vi "PostRegistration.vi"(8 "error in (no error)":errorcluster, 10 "state":T1(ring), 11 "VI ref":refnum<vi>) -> (0 "error out":errorcluster, 3 "VI ref":refnum<vi>)   [LabVIEW 2021, in "Autocomplete Textbox.lvlib"]
uses:
  Autocomplete Textbox.lvlib
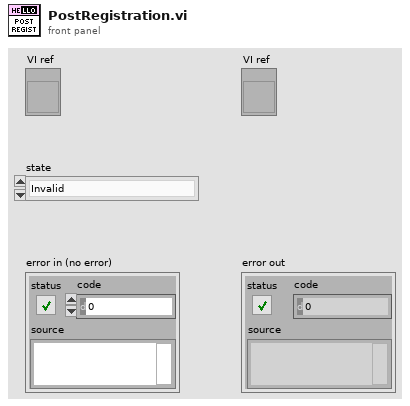
[diagram p1: front panel]
types:
  T1 = enum32{"Invalid", "Standard", "Closed", "Hidden", "Minimized", "Maximized"}
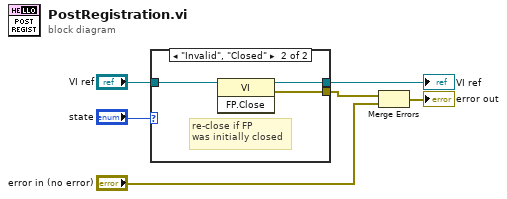
[diagram p0: block diagram]
diagram:
  n1 = case shown="\"Invalid\", \"Closed\"" "state" {
    tunnel: "VI ref" -> [w7 w10]
    tunnel: [_ w9] -> w6
    tunnel: [w7 w8] -> w2
    frame Default {
    }
    frame "Invalid", "Closed" {
      # "re-close if FP\nwas initially closed"
      n2 = invoke class="VI" method="FP.Close"(reference=w10) -> (reference out=w8:refnum<vi>, error out=w9:errorcluster)  [unwired: 2 in, 1 out]
    }
  }
  "VI ref" <- w2
  n3 = Merge Errors(w6, "error in (no error)") -> (→"error out":errorcluster)
